vi "jt_keithley-2450_python.vi"(0 "Scan settings":T2={"J-V scan"=TRUE, "Start voltage (V)"=0.0, "End voltage (V)"=0.0, "Step voltage (V)"=1.4, "Scan both directions"=TRUE, "Inverted device structure"=FALSE, "Measurement delay (ms)"=10.0, "Measurement speed"=0, "Scan rate (V/s)"=0.0, "Stabilisation time (s)"=0.0, "Stabilisation mode"=0, "Stabilisation value (V or A) "=1.0, "Illumination"=0, "Stabilisation in the dark?"=FALSE, "Repeat light scans"=FALSE, "No. of repeat scans"=0.0, "Only repeat for best pixel"=1, "J-t scan"=FALSE, "J-t best pixel only"=7, "J-t start voltage (V)"=0.0, "J-t end voltage (V)"=1.4, "J-t step voltage (V)"=0.01, "Step time (s)"=0.7, "J-t scan both directions"=TRUE, "J-t inverted device structure"=FALSE, "J-t settling delay (s)"=0.0, "J-t measurement speed"=0, "J-t illumination"=2, "Max. power stabilisation"=FALSE, "Max power best pixel only"=1, "Max. power point tracker"=FALSE, "Vmp from J-V scan"=FALSE, "Max P stab. Specific voltage"=FALSE, "Vmp (V)"=1.0, "Stabilisation time step (s)"=1.0, "Total stabilisation time (s)"=100.0} {"J-t settling delay (s)" min=0.0; "J-t illumination" items=["Light only", "Dark only", "Light then dark", "Dark then light"]; "Measurement speed" items=["Fast", "Normal", "High accuracy"]; "Illumination" items=["Light only", "Dark only", "Light then dark", "Dark then light"]; "Only repeat for best pixel" items=["only for best pixel", "for best 2 pixels", "for best 3 pixels", "for best 4 pixels", "for best 5 pixels", "for best 6 pixels", "for best 7 pixels", "for all pixels"]; "No. of repeat scans" min=1.0 step=1.0; "Max power best pixel only" items=["only the best pixel", "the best 2 pixels", "the best 3 pixels", "the best 4 pixels", "the best 5 pixels", "the best 6 pixels", "the best 7 pixels", "all pixels"]; "J-t best pixel only" items=["only the best pixel", "the best 2 pixels", "the best 3 pixels", "the best 4 pixels", "the best 5 pixels", "the best 6 pixels", "the best 7 pixels", "all pixels"]; "J-t measurement speed" items=["Fast", "Normal", "High Accuracy"]; "Stabilisation mode" items=["V", "I"]; "Measurement delay (ms)" min=10.0}, 1 "file name":string, 2 "folder path":string, 5 "Cell details cluster":T1={"Cell Position"=16, "Cell Label"="", "Pixel to measure"=0, "Area (cm^2)"=0.126, "Variable"="", "Variable value"="", "Scan settings in queue"=0, "Light or dark"="", "Measurement Type"=""} {"Pixel to measure" items=["All", "1", "2", "3", "4", "5", "6", "7", "8"]}, 11 "error in (no error)":errorcluster, 12 "illumination intensity (suns equiv.)":string) -> (15 "error out":errorcluster)   [LabVIEW 2016]
uses:
  TypeDefs/scan_settings.ctl
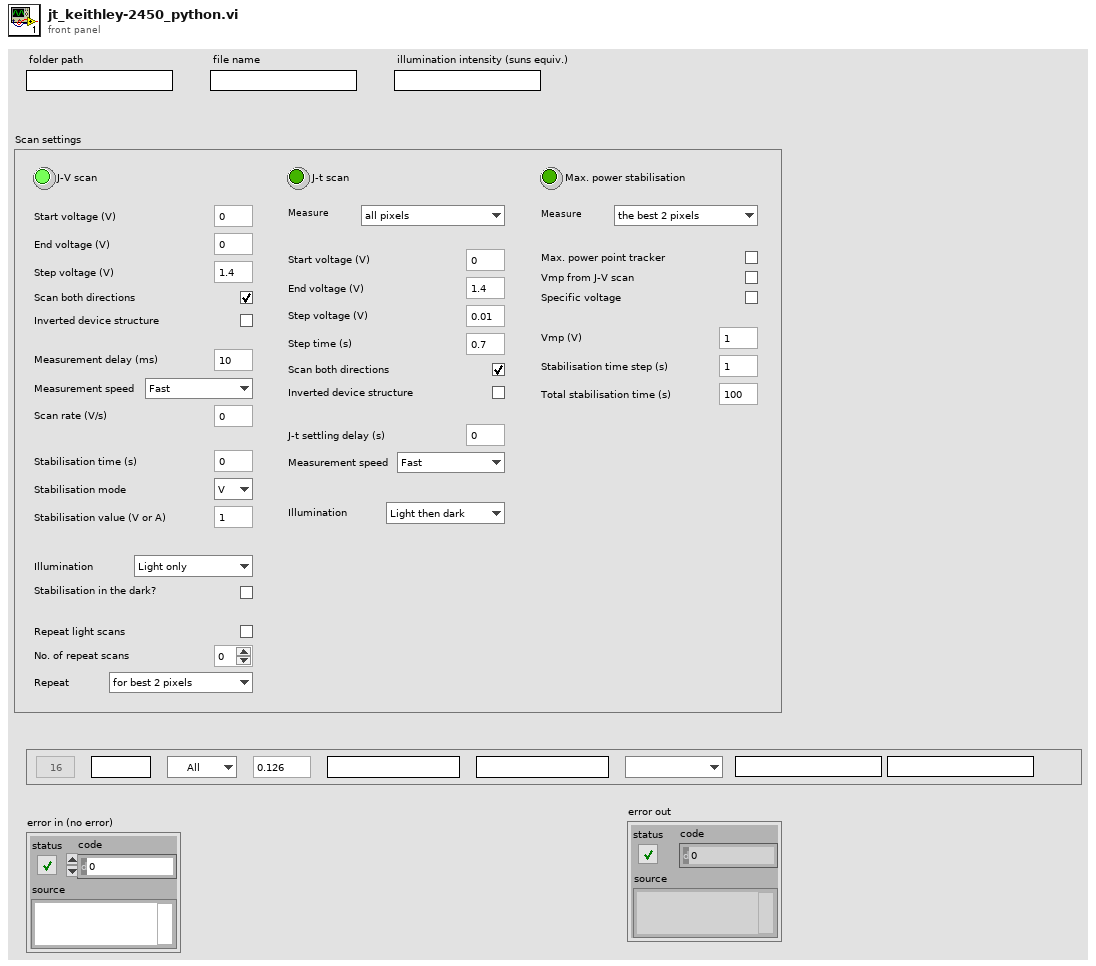
[diagram p1: front panel]
types:
  T1 = cluster{"Cell Position":i32, "Cell Label":string, "Pixel to measure":u16, "Area (cm^2)":dbl, "Variable":string, "Variable value":string, "Scan settings in queue":u16, "Light or dark":string, "Measurement Type":string}
  T2 = typedef "scan_settings.ctl" = cluster{"J-V scan":bool, "Start voltage (V)":dbl, "End voltage (V)":dbl, "Step voltage (V)":dbl, "Scan both directions":bool, "Inverted device structure":bool, "Measurement delay (ms)":dbl, "Measurement speed":u8, "Scan rate (V/s)":dbl, "Stabilisation time (s)":dbl, "Stabilisation mode":u16, "Stabilisation value (V or A) ":dbl, "Illumination":u16, "Stabilisation in the dark?":bool, "Repeat light scans":bool, "No. of repeat scans":dbl, "Only repeat for best pixel":u16, "J-t scan":bool, "J-t best pixel only":u16, "J-t start voltage (V)":dbl, "J-t end voltage (V)":dbl, "J-t step voltage (V)":dbl, "Step time (s)":dbl, "J-t scan both directions":bool, "J-t inverted device structure":bool, "J-t settling delay (s)":dbl, "J-t measurement speed":u16, "J-t illumination":u16, "Max. power stabilisation":bool, "Max power best pixel only":u16, "Max. power point tracker":bool, "Vmp from J-V scan":bool, "Max P stab. Specific voltage":bool, "Vmp (V)":dbl, "Stabilisation time step (s)":dbl, "Total stabilisation time (s)":dbl}
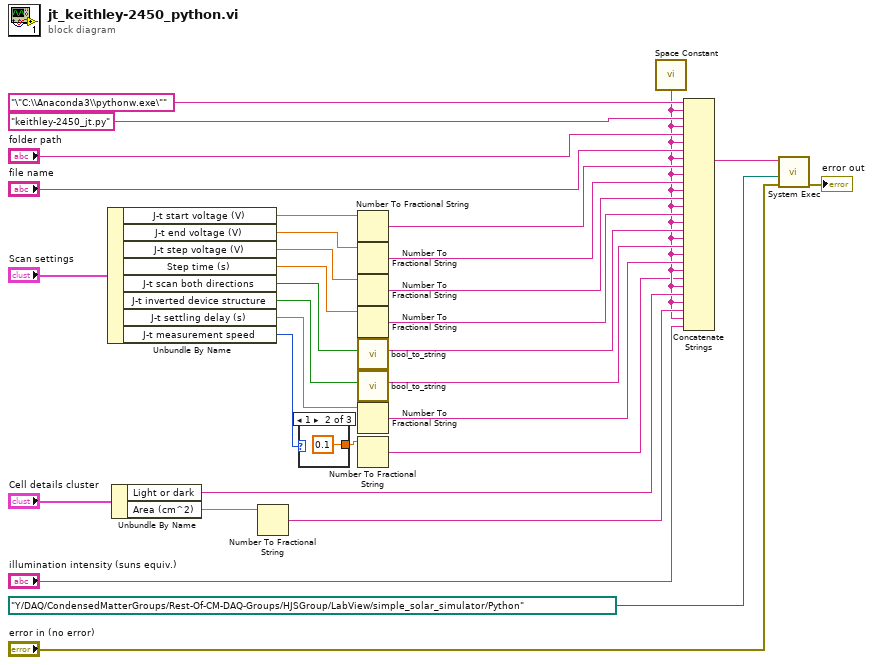
[diagram p0: block diagram]
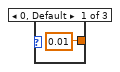
[diagram p2: hidden frame]
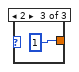
[diagram p3: hidden frame]
diagram:
  n1 = Unbundle By Name("Scan settings") -> ("J-t start voltage (V)"=w22:dbl, "J-t end voltage (V)"=w21:dbl, "J-t step voltage (V)"=w20:dbl, "Step time (s)"=w19:dbl, "J-t scan both directions"=w18:bool, "J-t inverted device structure"=w17:bool, "J-t settling delay (s)"=w16:dbl, "J-t measurement speed"=w14:u16)
  n2 = Unbundle By Name("Cell details cluster") -> ("Light or dark"=w4:string, "Area (cm^2)"=w5:dbl)
  n3 = Number To Fractional String(number=w5) -> (F-format string=w3:string)  [unwired: 3 in]
  n4 = case shown="1" w14 {
    tunnel: [0.01 0.1 1] -> w15
    frame 0, Default {
    }
    frame 1 {
    }
    frame 2 {
    }
  }
  n5 = Number To Fractional String(number=w22) -> (F-format string=w12:string)  [unwired: 3 in]
  n6 = Number To Fractional String(number=w21) -> (F-format string=w11:string)  [unwired: 3 in]
  n7 = Number To Fractional String(number=w20) -> (F-format string=w10:string)  [unwired: 3 in]
  n8 = Number To Fractional String(number=w19) -> (F-format string=w9:string)  [unwired: 3 in]
  n9 = call "bool_to_string.vi"("Boolean"=w18) -> ("String"=w8:string)  [unwired: 10 in]
  n10 = call "bool_to_string.vi"("Boolean"=w17) -> ("String"=w7:string)  [unwired: 10 in]
  n11 = Number To Fractional String(number=w16) -> (F-format string=w6:string)  [unwired: 3 in]
  n12 = Number To Fractional String(number=w15) -> (F-format string=w1:string)  [unwired: 3 in]
  n13 = call <vilib>:"Space Constant.vi"() -> ("String"=w2:string)
  n14 = Concatenate Strings("\"C:\\Anaconda3\\pythonw.exe\"" ("standard input"), w2, "keithley-2450_jt.py" ("standard input"), w2, "folder path", w2, "file name", w2, w12, w2, w11, w2, w10, w2, w9, w2, w8, w2, w7, w2, w6, w2, w1, w2, w4, w2, w3, w2, "illumination intensity (suns equiv.)") -> (w30:string)
  n15 = call <vilib>:"System Exec.vi"("error in (no error)"="error in (no error)", "working directory"=path "Y:/DAQ/CondensedMatterGroups/Rest-Of-CM-DAQ-Groups/HJSGroup/LabView/simple_solar_simulator/Python", "command line"=w30) -> ("error out"=→"error out":errorcluster)  [unwired: 5 in, 3 out]
